vi "Calibrate Zero Volts to all channels.vi"(5 "Device Name":string) -> (0 "error out":errorcluster, 2 "Return Code":i32, 3 "Report Text":string)   [LabVIEW 2015]
uses:
  DAQ/Relay Modes.ctl
  DAQ/Channels_v2.ctl
panel:
  in  "error in (no error)":errorcluster
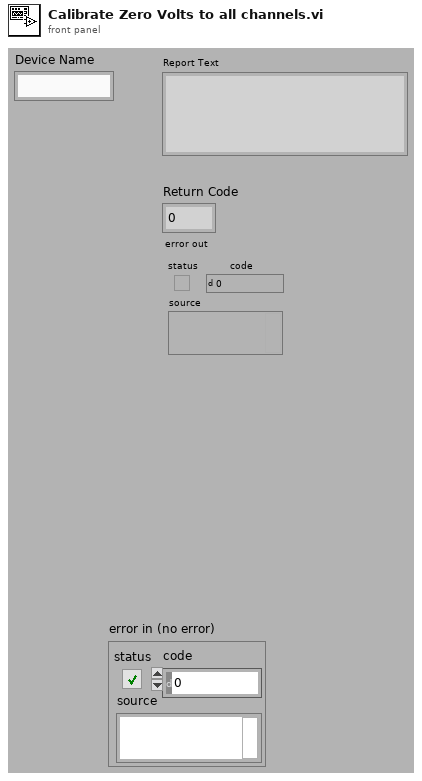
[diagram p1: front panel]
types:
  T1 = typedef "Channels_v2.ctl" = enum16{"All Off", "Channel 4", "Channel 3", "4,3", "Channel 2", "4,2", "3,2", "4,3,2,", "Channel 1", "4,1", "3,1", "4,3,1", "2,1", "4,2,1", "3,2,1", "All On"}
  T2 = typedef "Relay Modes.ctl" = enum16{"All Off", "Short", "Ohms", "Fluke", "Daq AO 0"}
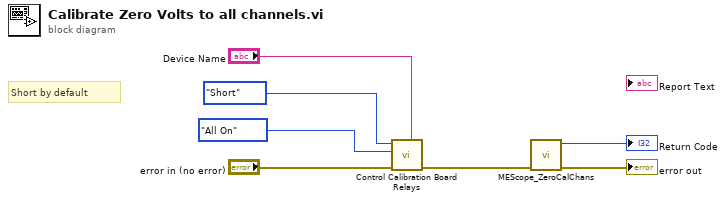
[diagram p0: block diagram]
diagram:
  # "Short by default"
  n1 = call "Control Calibration Board Relays.vi"("Device Name"="Device Name", "error in"="error in (no error)", "Channels"=Channels_v2."All On", "Mode"=Relay_Modes."Short") -> ("error out"=w5:errorcluster)  [unwired: 7 in]
  n2 = call "MEScope_ZeroCalChans.vi"("error in"=w5) -> ("error out"=→"error out":errorcluster, "Return Code"=→"Return Code":i32)  [unwired: 9 in]
